vi "Create Datalog w header.vi"(8 "error in":errorcluster) -> (0 "error out":errorcluster, 1 "Valid File":bool, 2 "path":path, 3 "File refnum":refnum<file>)   [LabVIEW 2010]
doc: "Closes the previous File reference.\nOpens or creates a new File.\nSave a header based on the global variable Calibration matrix.\nThe File reference is an output that can be used by the datalogger.vi"
uses:
  calibration/global scale array.vi
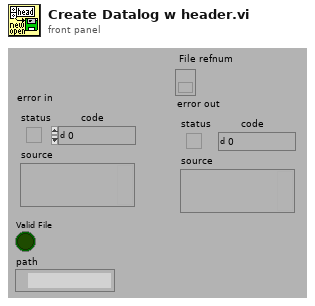
[diagram p1: front panel]
types:
  T1 = typedef "calib array.ctl" = T2[]
  T2 = typedef "conversion.ctl" = cluster{"conversion matrix":sgl[][], "units":string, "name":string, "scale type":T3, "offset (volts)":dbl, "second channel":i8, "correspondence table":T4, "offset (physical units)":dbl, "pH scale":T5, "D.O.":T6}
  T3 = typedef "scale type.ctl" = enum16{"Volts", "Polynomial", "Correspondence Table", "pH", "Dissolved Oxygen", "Quadratic"}
  T4 = typedef "correspondence table.ctl" = cluster{"physical units":dbl, "volts":dbl}[]
  T5 = typedef "pH scale.ctl" = cluster{"Buffers":cluster{"Buffer":dbl, "Calibrated":bool, "V/T":dbl}[], "Temperature":dbl}
  T6 = typedef "DO scale.ctl" = cluster{"Temperature":dbl, "K":dbl, "barometric pressure":dbl}
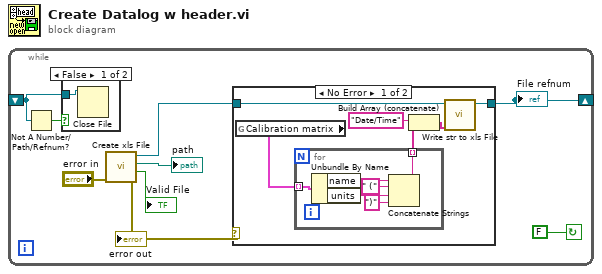
[diagram p0: block diagram]
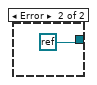
[diagram p3: hidden frame]
diagram:
  n1 = while {
    shift-left: _ -> [w2]
    shift-right: [w7] -> _
    stop <- FALSE continue-if-true
    n2 = Not A Number/Path/Refnum?(number/path/refnum=w2) -> (NaN/Path/Refnum?=w5:bool)
    n3 = case shown="False" w5 {
      tunnel: w2 -> [w10 _]
      frame False {
        n4 = Close File(refnum=w10) -> ()  [unwired: 1 in, 2 out]
      }
      frame True {
      }
    }
    n5 = call "Create xls File.vi"("error in"="error in") -> ("error out"=w8:errorcluster, "Valid File"=→"Valid File":bool, "path"=→"path":path, "refnum"=w9:refnum<file>)  [unwired: 3 in]
    "error out" <- w8
    n6 = case shown="No Error" w8 {
      tunnel: w9 -> [w16 _]
      tunnel: [w11 refnum<k0> refnum] -> w7
      frame No Error {
        n7 = global read "global scale array.vi" "Calibration matrix"() -> (w15:T1)
        n8 = for {
          tunnel: w15 -> [w22] mode=indexing
          tunnel: [w20] -> w14 mode=indexing
          n9 = Unbundle By Name(w22) -> ("name"=w21:string, "units"=w19:string)
          n10 = Concatenate Strings(w21, " (" ("Substring"), w19, ")" ("Substring")) -> (w20:string)
        }
        n11 = Build Array (concatenate)("Date/Time" ("Substring"), w14) -> (w13:string[])
        n12 = call "Write str to xls File.vi"("error in (no error)"=w13, "refnum"=w16) -> ("dup refnum"=w11:refnum<file>)  [unwired: 8 in, 1 out]
      }
      frame Error {
      }
    }
    "File refnum" <- w7
  }
